vi "DAQ_Digital Clk Gen Configure and Generate.vi"(0 "DAQmx Task In":refnum<k21>, 5 "Digital Clock Settings":T2={"Frequency (Hz)"=10000.0, "Duty Cycle(%)"=50.0, "Generation Time (s)"=0.1} {"Duty Cycle(%)" format="%#.2p"; "Frequency (Hz)" format="%.6p"; "Generation Time (s)" format="%.2p"}, 11 "error in":errorcluster) -> (4 "DAQmx Task Out":refnum<k21>, 6 "Actual Clock Settings":T1={"Frequency (Hz)"=10000.0, "Duty Cycle (%)"=50.0, "Generation Time (s)"=0.1} {"Duty Cycle (%)" format="%#.2p"; "Frequency (Hz)" format="%.6p"; "Generation Time (s)" format="%.2p"}, 15 "error out":errorcluster)   [LabVIEW 2021, in "DAQ_Digital Clock Generation.lvlib"]
doc: "Configure and Generate Digital pulses in the configured terminal using Counters"
uses:
  DAQ_Digital Clock Generation.lvlib
  Typedefs/Digital Clock Settings.ctl
  Typedefs/Actual Clock Settings.ctl
  <vilib>/DAQmx/configure/timing.llb/DAQmx Timing (Implicit).vi
  <resource>/objmgr/daqmx.rc
panel:
  out "Timebase Frequency (Hz)":dbl=80000000.0 format="%#.6p"
  # "Outputs"
  # "Inputs"
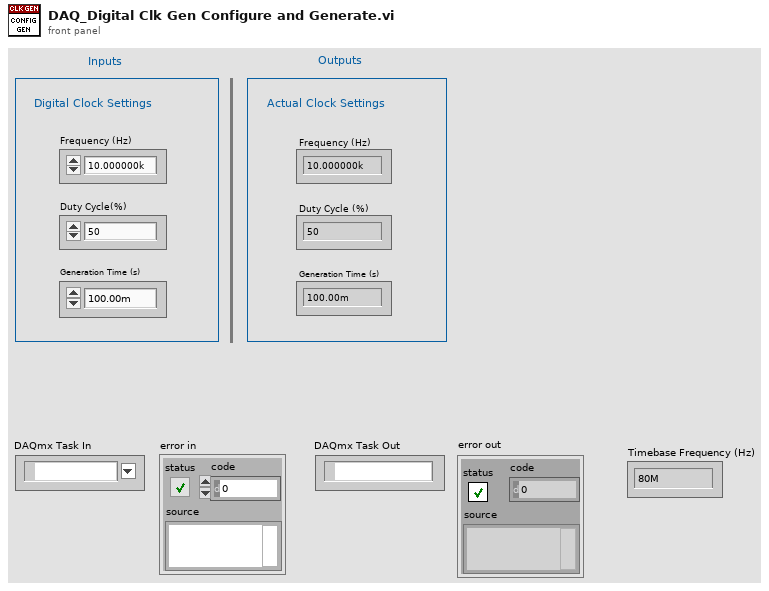
[diagram p1: front panel]
types:
  T1 = typedef "DAQ_Digital Clock Generation.lvlib/Actual Clock Settings.ctl" = cluster{"Frequency (Hz)":dbl, "Duty Cycle (%)":dbl, "Generation Time (s)":dbl}
  T2 = typedef "DAQ_Digital Clock Generation.lvlib/Digital Clock Settings.ctl" = cluster{"Frequency (Hz)":dbl, "Duty Cycle(%)":dbl, "Generation Time (s)":dbl}
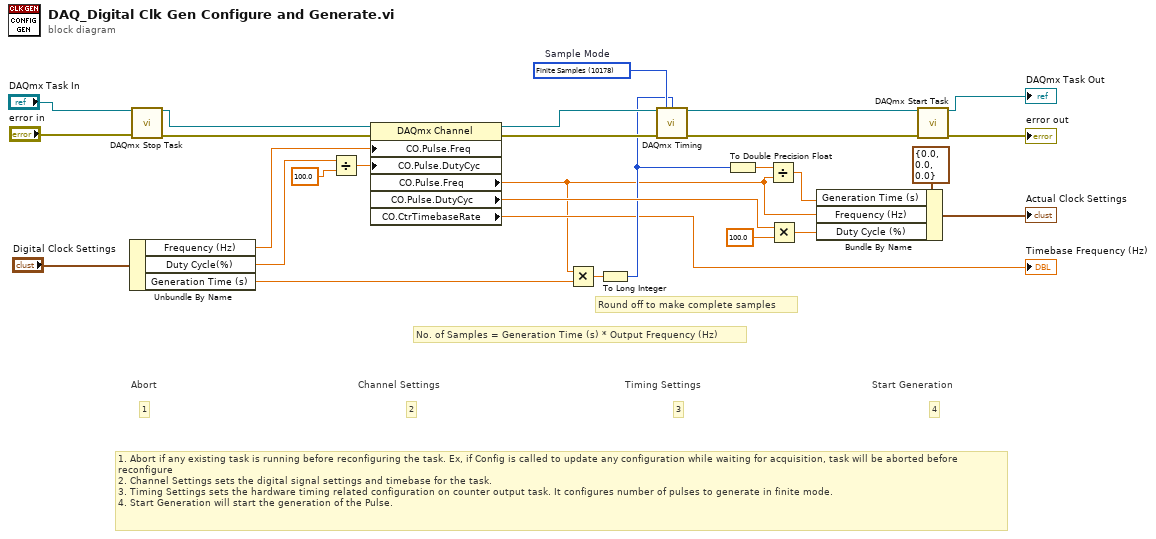
[diagram p0: block diagram]
diagram:
  w24 = 10178 items=["Finite Samples"=10178, "Continuous Samples"=10123, "Hardware Timed Single Point"=12522]  # Sample Mode
  # "Round off to make complete samples"
  # "No. of Samples = Generation Time (s) * Output Frequency (Hz)"
  # "1"
  # "4"
  # "3"
  # "2"
  # "Abort"
  # "1. Abort if any existing task is running before reconfiguring the task. Ex, if Config is called to update any configuration while waiting for acquisition, task will be aborted before reconfigure\n2. Channel Settings sets the digital signal settings and timebase for the task.\n3. Timing Settings sets the hardware timing related configuration on counter output task. It configures number of pulses to generate in finite mode.\n4. Start Generation will start the generation of the Pulse."
  # "Start Generation"
  # "Timing Settings"
  # "Channel Settings"
  n1 = Unbundle By Name("Digital Clock Settings") -> ("Frequency (Hz)"=w3:dbl, "Duty Cycle(%)"=w4:dbl, "Generation Time (s)"=w16:dbl)
  n2 = call <vilib>:"DAQmx Stop Task.vi"("task/channels in"="DAQmx Task In", "error in"="error in") -> ("task out"=w19:refnum<k21>, "error out"=w18:errorcluster)  [unwired: 12 in]
  n3 = Divide(x=w4, y=100.0) -> (x/y=w11:dbl)
  n4 = property class="DAQmx Channel"(reference=w19, error in=w18, "CO.Pulse.Freq"=w3, "CO.Pulse.DutyCyc"=w11) -> (reference out=w27:refnum<k21>, error out=w28:errorcluster, "CO.Pulse.Freq"=w1:dbl, "CO.Pulse.DutyCyc"=w8:dbl, "CO.CtrTimebaseRate"=→"Timebase Frequency (Hz)":dbl)
  n5 = Multiply(x=w1, y=w16) -> (x*y=w6:dbl)
  n6 = To Long Integer(number=w6) -> (32bit integer=w5:i32)
  n7 = call-poly <vilib>:"DAQmx Timing.vi"("task/channels in"=w27, "sample mode"=w24, "samples per channel"=w5, "error in"=w28) -> ("task out"=w17:refnum<k21>, "error out"=w26:errorcluster)  [unwired: 10 in]
  n8 = To Double Precision Float(number=w5) -> (double precision float=w12:dbl)
  n9 = Divide(x=w12, y=w1) -> (x/y=w13:dbl)
  n10 = Multiply(x=w8, y=100.0) -> (x*y=w9:dbl)
  n11 = Bundle By Name(cluster=T1 {"Frequency (Hz)"=0.0, "Duty Cycle (%)"=0.0, "Generation Time (s)"=0.0} ("Actual Pulse Settings"), "Generation Time (s)"=w13, "Frequency (Hz)"=w1, "Duty Cycle (%)"=w9) -> (→"Actual Clock Settings":T1)
  n12 = call <vilib>:"DAQmx Start Task.vi"("task/channels in"=w17, "error in"=w26) -> ("task out"=→"DAQmx Task Out":refnum<k21>, "error out"=→"error out":errorcluster)  [unwired: 12 in]
